vi "Auto settings.vi"(8 "error in (no error)":errorcluster, 10 "Assembly Settings":T1, 11 "Syringe Space in":refnum<class "Syringe Space.lvclass">) -> (0 "error out":errorcluster, 3 "Syringe Space out":refnum<class "Syringe Space.lvclass">)   [LabVIEW 2021, in "Syringe Space.lvclass"]
uses:
  Syringe Space.lvclass
  C:/Users/HEP/Documents/GitHub/Gantry/UCSB-Gantry-HEP-main/Classes/Workspace/Fixture.lvclass
  C:/Users/HEP/Documents/GitHub/Gantry/UCSB-Gantry-HEP-main/Classes/Workspace/Carrier Tray/Assembly Tray.lvclass
  Fixture.lvclass/Fixture.ctl
  Assembly Tray.lvclass/Assembly Tray.ctl
  Write Fixture ID.vi
  Write Syringe.vi
  Write Gantry Region.vi
  Write Position.vi
  SubVIs/assembly_tray_region.vi
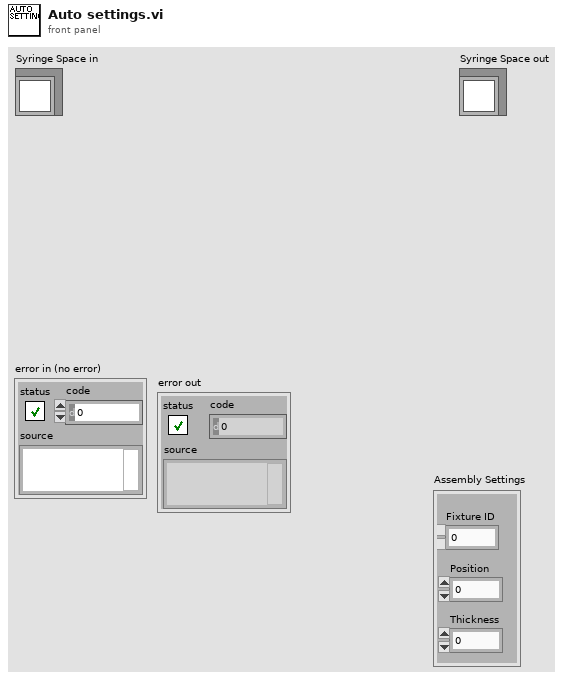
[diagram p1: front panel]
types:
  T1 = cluster{"Fixture ID":dbl, "Position":dbl, "Thickness":dbl}
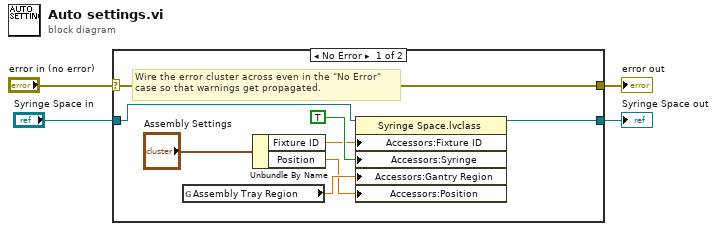
[diagram p0: block diagram]
diagram:
  n1 = case shown="No Error" "error in (no error)" {
    selector: "error in (no error)" -> [w12 w14]
    tunnel: [w12 w14] -> w3
    tunnel: [w9 w13] -> w1
    tunnel: "Syringe Space in" -> [w10 w13]
    frame No Error {
      # "Wire the error cluster across even in the \"No Error\"\ncase so that warnings get propagated."
      n2 = global read "assembly_tray_region.vi" "Assembly Tray Region"() -> (w8:dbl)
      n3 = Unbundle By Name("Assembly Settings") -> ("Fixture ID"=w7:dbl, "Position"=w6:dbl)
      n4 = property class="Syringe Space.lvclass"(reference=w10, "Accessors:Fixture ID"=w7, "Accessors:Syringe"=TRUE ("Syringe"), "Accessors:Gantry Region"=w8, "Accessors:Position"=w6) -> (reference out=w9:refnum<class "Syringe Space.lvclass">)  [unwired: 1 in, 1 out]
    }
    frame Error {
    }
  }
  "error out" <- w3
  "Syringe Space out" <- w1
